vi "cloneXML.vi"(8 "error in (no error)":errorcluster, 11 "NativeXML in":refnum<class "NativeXML.lvclass">) -> (0 "error out":errorcluster, 2 "NativeXML clone":refnum<class "NativeXML.lvclass">, 3 "NativeXML out":refnum<class "NativeXML.lvclass">)   [LabVIEW 2011, in "Tools.lvlib" / "xml.lvlib" / "NativeXML.lvclass"]
uses:
  NativeXML.lvclass
  NativeXML.lvclass/NativeXML.ctl
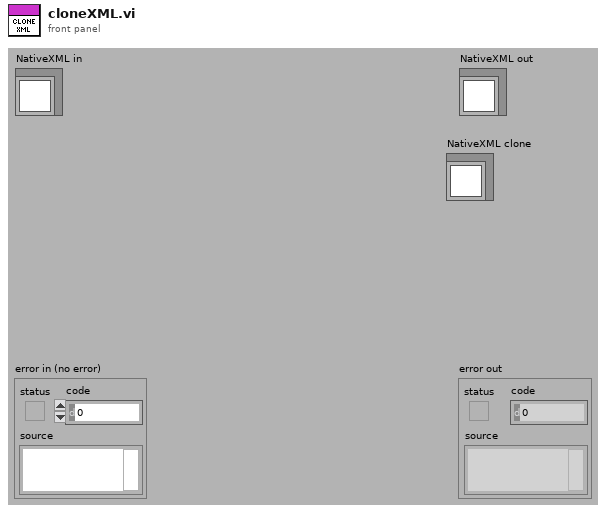
[diagram p1: front panel]
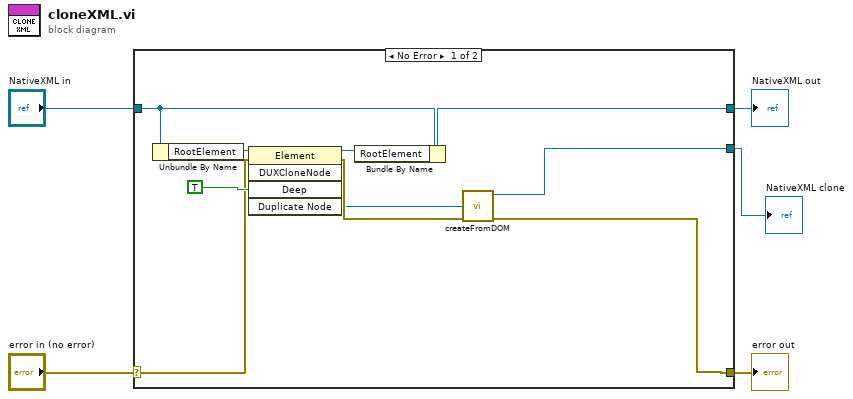
[diagram p0: block diagram]
diagram:
  n1 = case shown="No Error" "error in (no error)" {
    selector: "error in (no error)" -> [w10 w17]
    tunnel: [w14 w17] -> w4
    tunnel: [w7 w16] -> w2
    tunnel: "NativeXML in" -> [w8 w16]
    tunnel: [w15 _] -> w1
    frame No Error {
      n2 = Unbundle By Name(w8) -> ("RootElement"=w13:refnum<k20>)
      n3 = invoke class="Element" method="DUXCloneNode"(reference=w13, error in=w10, "Deep"=TRUE) -> (reference out=w9:refnum<k20>, error out=w11:errorcluster, "Duplicate Node"=w6:refnum<k20>)  [unwired: 2 in, 2 out]
      n4 = Bundle By Name(cluster=w8, "RootElement"=w9) -> (w7:refnum<class "NativeXML.lvclass">)
      n5 = call "createFromDOM.vi"("error in (no error)"=w11, "RootElement"=w6) -> ("error out"=w14:errorcluster, "NativeXML out"=w15:refnum<class "NativeXML.lvclass">)  [unwired: 8 in]
    }
    frame Error {
    }
  }
  "error out" <- w4
  "NativeXML out" <- w2
  "NativeXML clone" <- w1
